vi "GLB_PID.vi"() -> ()   [LabVIEW 2014, in "PLS Generation.lvlib"]
uses:
  PLS Generation.lvlib
  <userlib>/_MGI/Numeric/MGI Handle PID State Cluster.ctl
panel:
  out "last re-init":timestamp
  in  "state":T1
  in  "PID":cluster{"P":dbl, "I":dbl, "D":dbl}
  in  "PID actif":bool
  in  "output":dbl
  in  "output PID":dbl
  in  "input":dbl
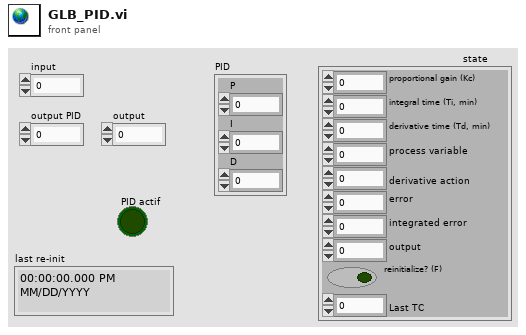
[diagram p1: front panel]
types:
  T1 = typedef "MGI Handle PID State Cluster.ctl" = cluster{"proportional gain (Kc)":dbl, "integral time (Ti, min)":dbl, "derivative time (Td, min)":dbl, "process variable":dbl, "derivative action":dbl, "error":dbl, "integrated error":dbl, "output":dbl, "reinitialize? (F)":bool, "Last TC":u32}
diagram:
